vi "filter_app.vi"() -> ()   [LabVIEW 2012, in "LightPipes.lvlib"]
uses:
  LightPipes.lvlib
panel:
  in  "c2":i16(ring) items=["subst", "mult"]
  in  "c1":i16(ring) items=["int", "pha"]
  out "Field out":cluster{"n_grid":i32, "size":dbl, "lambda":dbl}
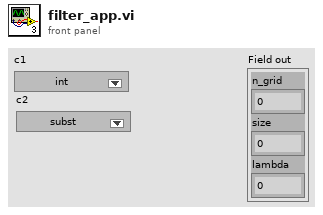
[diagram p1: front panel]
types:
  T1 = cluster{"n_grid":i32, "@dummy control@":i8, "@dummy control@":i8, "@dummy control@":i8, "@dummy control@":i8, "size":dbl, "lambda":dbl, "int1":i32, "int2":i32, "int3":i32, "@dummy control@":i8, "@dummy control@":i8, "@dummy control@":i8, "@dummy control@":i8, "double1":dbl, "double2":dbl, "double3":dbl, "real":u32, "imaginary":u32}
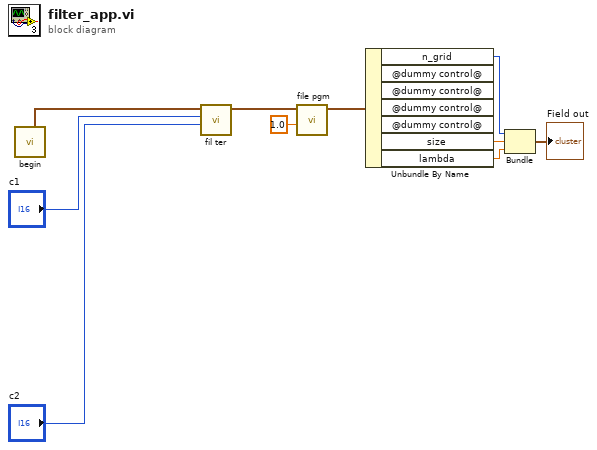
[diagram p0: block diagram]
diagram:
  n1 = call "begin.vi"() -> ("field out"=w5:T1)  [unwired: 11 in]
  n2 = call "fil ter.vi"("multiplication/ substitution"="c2", "intensity / phase"="c1", "field"=w5) -> ("field out"=w4:T1)  [unwired: 7 in, 1 out]
  n3 = call "file pgm.vi"("gamma"=1.0, "field"=w4) -> ("field out"=w6:T1)  [unwired: 8 in, 1 out]
  n4 = Unbundle By Name(w6) -> ("n_grid"=w7:i32, "size"=w8:dbl, "lambda"=w9:dbl)  [unwired: 4 out]
  n5 = Bundle("n_grid"=w7, "size"=w8, "lambda"=w9) -> (→"Field out":cluster{"n_grid":i32, "size":dbl, "lambda":dbl})  [unwired: 1 in]
